vi "公式写入.vi"(7 "公式":cluster{"X^2":dbl, "X":dbl, "b":dbl}, 8 "error in (no error)":errorcluster caption="错误输入（无错误）", 9 "量程":enum16{"低量程", "高量程"}(ring), 10 "测量模式":enum16{"水样测量", "零点核查", "跨度核查", "标样核查", "加标回收"}(ring), 11 "测量参数":enum16{"总磷", "总氮", "氨氮"}(ring)) -> (0 "error out":errorcluster caption="错误输出")   [LabVIEW 2016, in "斯坦道氨氮.lvlib"]
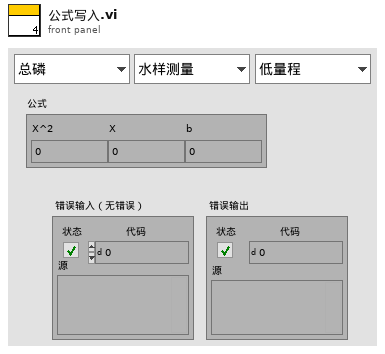
[diagram p1: front panel]
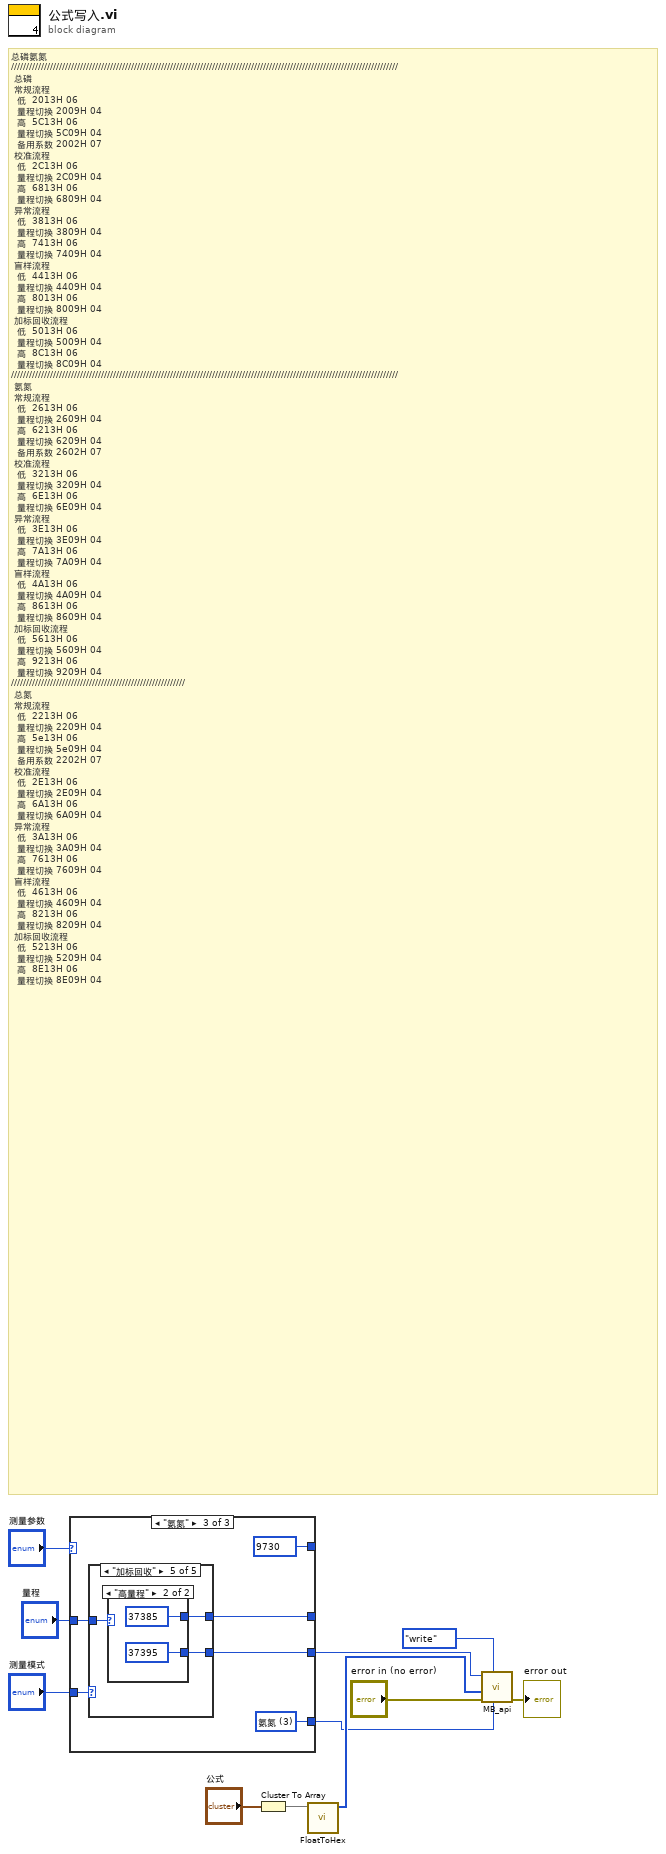
[diagram p0: block diagram]
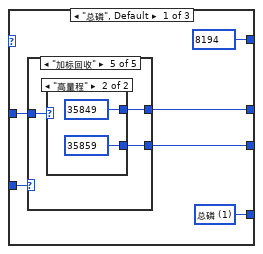
[diagram p2: hidden frame]
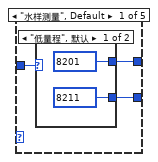
[diagram p3: hidden frame]
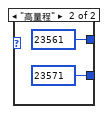
[diagram p4: hidden frame]
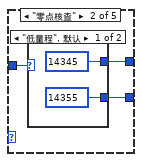
[diagram p5: hidden frame]
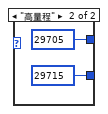
[diagram p6: hidden frame]
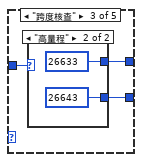
[diagram p7: hidden frame]
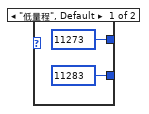
[diagram p8: hidden frame]
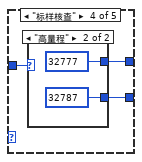
[diagram p9: hidden frame]
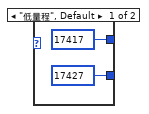
[diagram p10: hidden frame]
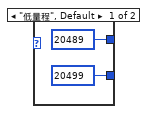
[diagram p11: hidden frame]
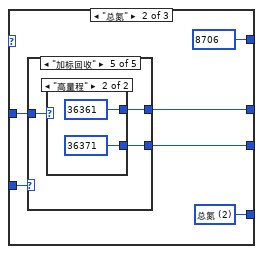
[diagram p12: hidden frame]
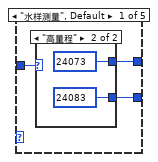
[diagram p13: hidden frame]
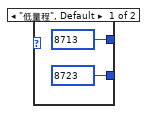
[diagram p14: hidden frame]
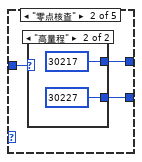
[diagram p15: hidden frame]
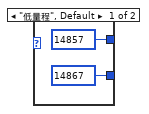
[diagram p16: hidden frame]
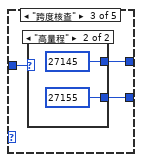
[diagram p17: hidden frame]
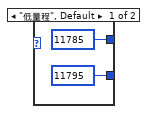
[diagram p18: hidden frame]
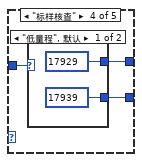
[diagram p19: hidden frame]
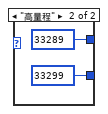
[diagram p20: hidden frame]
diagram:
  # "总磷氨氮\n/////////////////////////////////////////////////////////////////////////////////////////////////////////////////////////////////\n\t总磷\n\t常规流程\n\t\t低\t\t2013H\t06\n\t\t量程切换\t2009H\t04\n\t\t高\t\t5C13H\t06\n\t\t量程切换\t5C09H\t04\n\t\t备用系数\t2002H\t07\n\t校准流程\n\t\t低\t\t2C13H\t06\n\t\t量程切换\t2C09H\t04\n\t\t高\t\t6813H\t06\n\t\t量程切换\t6809H\t04\n\t异常流程\n\t\t低\t\t3813H\t06\n\t\t量程切换\t3809H\t04\n\t\t高\t\t7413H\t06\n\t\t量程切换\t7409H\t04\t\n\t盲样流程\n\t\t低\t\t4413H\t06\n\t\t量程切换\t4409H\t04\n\t\t高\t\t8013H\t06\n\t\t量程切换\t8009H\t04\t\n\t加标回收流程\n\t\t低\t\t5013H\t06\n\t\t量程切换\t5009H\t04\n\t\t高\t\t8C13H\t06\n\t\t量程切换\t8C09H\t04\t\n/////////////////////////////////////////////////////////////////////////////////////////////////////////////////////////////////\n\t氨氮\n\t常规流程\n\t\t低\t\t2613H\t06\n\t\t量程切换\t2609H\t04\n\t\t高\t\t6213H\t06\n\t\t量程切换\t6209H\t04\n\t\t备用系数\t2602H\t07\n\t校准流程\n\t\t低\t\t3213H\t06\n\t\t量程切换\t3209H\t04\n\t\t高\t\t6E13H\t06\n\t\t量程切换\t6E09H\t04\n\t异常流程\n\t\t低\t\t3E13H\t06\n\t\t量程切换\t3E09H\t04\n\t\t高\t\t7A13H\t06\n\t\t量程切换\t7A09H\t04\t\n\t盲样流程\n\t\t低\t\t4A13H\t06\n\t\t量程切换\t4A09H\t04\n\t\t高\t\t8613H\t06\n\t\t量程切换\t8609H\t04\t\n\t加标回收流程\n\t\t低\t\t5613H\t06\n\t\t量程切换\t5609H\t04\n\t\t高\t\t9213H\t06\n\t\t量程切换\t9209H\t04\t\n//////////////////////////////////////////////////////////\n\t总氮\n\t常规流程\n\t\t低\t\t2213H\t06\n\t\t量程切换\t2209H\t04\n\t\t高\t\t5e13H\t06\n\t\t量程切换\t5e09H\t04\n\t\t备用系数\t2202H\t07\n\t校准流程\n\t\t低\t\t2E13H\t06\n\t\t量程切换\t2E09H\t04\n\t\t高\t\t6A13H\t06\n\t\t量程切换\t6A09H\t04\n\t异常流程\n\t\t低\t\t3A13H\t06\n\t\t量程切换\t3A09H\t04\n\t\t高\t\t7613H\t06\n\t\t量程切换\t7609H\t04\t\n\t盲样流程\n\t\t低\t\t4613H\t06\n\t\t量程切换\t4609H\t04\n\t\t高\t\t8213H\t06\n\t\t量程切换\t8209H\t04\t\n\t加标回收流程\n\t\t低\t\t5213H\t06\n\t\t量程切换\t5209H\t04\n\t\t高\t\t8E13H\t06\n\t\t量程切换\t8E09H\t04"
  n1 = case shown="\"氨氮\"" "测量参数" {
    tunnel: "测量模式" -> [w17 w58 w99]
    tunnel: "量程" -> [w16 w57 w98]
    tunnel: [w15 w56 w97] -> w1
    tunnel: [w14 w55 w96] -> w8
    tunnel: [w13 w54 w95] -> _
    tunnel: [u16 8194 ("starting address") u16 8706 ("starting address") u16 9730 ("starting address")] -> _
    frame "总磷", Default {
      w15 = u16 1 items=["总磷"=1, "氨氮"=3] ("站号")
      n2 = case shown="\"加标回收\"" w17 {
        tunnel: w16 -> [w20 w27 w34 w41 w48]
        tunnel: [w19 w26 w33 w40 w47] -> w14
        tunnel: [w18 w25 w32 w39 w46] -> w13
        frame "水样测量", Default {
          n3 = case shown="\"低量程\", 默认" w20 {
            tunnel: [u16 8211 ("starting address") u16 23571 ("starting address")] -> w19
            tunnel: [u16 8201 ("starting address") u16 23561 ("starting address")] -> w18
            frame "低量程", Default {
            }
            frame "高量程" {
            }
          }
        }
        frame "零点核查" {
          n4 = case shown="\"低量程\", 默认" w27 {
            tunnel: [u16 14355 ("starting address") u16 29715 ("starting address")] -> w26
            tunnel: [u16 14345 ("starting address") u16 29705 ("starting address")] -> w25
            frame "低量程", Default {
            }
            frame "高量程" {
            }
          }
        }
        frame "跨度核查" {
          n5 = case shown="\"高量程\"" w34 {
            tunnel: [u16 11283 ("starting address") u16 26643 ("starting address")] -> w33
            tunnel: [u16 11273 ("starting address") u16 26633 ("starting address")] -> w32
            frame "低量程", Default {
            }
            frame "高量程" {
            }
          }
        }
        frame "标样核查" {
          n6 = case shown="\"高量程\"" w41 {
            tunnel: [u16 17427 ("starting address") u16 32787 ("starting address")] -> w40
            tunnel: [u16 17417 ("starting address") u16 32777 ("starting address")] -> w39
            frame "低量程", Default {
            }
            frame "高量程" {
            }
          }
        }
        frame "加标回收" {
          n7 = case shown="\"高量程\"" w48 {
            tunnel: [u16 20499 ("starting address") u16 35859 ("starting address")] -> w47
            tunnel: [u16 20489 ("starting address") u16 35849 ("starting address")] -> w46
            frame "低量程", Default {
            }
            frame "高量程" {
            }
          }
        }
      }
    }
    frame "总氮" {
      w56 = u16 2 items=["总磷"=1, "总氮"=2, "氨氮"=3] ("站号")
      n8 = case shown="\"加标回收\"" w58 {
        tunnel: w57 -> [w61 w68 w75 w82 w89]
        tunnel: [w60 w67 w74 w81 w88] -> w55
        tunnel: [w59 w66 w73 w80 w87] -> w54
        frame "水样测量", Default {
          n9 = case shown="\"高量程\"" w61 {
            tunnel: [u16 8723 ("starting address") u16 24083 ("starting address")] -> w60
            tunnel: [u16 8713 ("starting address") u16 24073 ("starting address")] -> w59
            frame "低量程", Default {
            }
            frame "高量程" {
            }
          }
        }
        frame "零点核查" {
          n10 = case shown="\"高量程\"" w68 {
            tunnel: [u16 14867 ("starting address") u16 30227 ("starting address")] -> w67
            tunnel: [u16 14857 ("starting address") u16 30217 ("starting address")] -> w66
            frame "低量程", Default {
            }
            frame "高量程" {
            }
          }
        }
        frame "跨度核查" {
          n11 = case shown="\"高量程\"" w75 {
            tunnel: [u16 11795 ("starting address") u16 27155 ("starting address")] -> w74
            tunnel: [u16 11785 ("starting address") u16 27145 ("starting address")] -> w73
            frame "低量程", Default {
            }
            frame "高量程" {
            }
          }
        }
        frame "标样核查" {
          n12 = case shown="\"低量程\", 默认" w82 {
            tunnel: [u16 17939 ("starting address") u16 33299 ("starting address")] -> w81
            tunnel: [u16 17929 ("starting address") u16 33289 ("starting address")] -> w80
            frame "低量程", Default {
            }
            frame "高量程" {
            }
          }
        }
        frame "加标回收" {
          n13 = case shown="\"高量程\"" w89 {
            tunnel: [u16 21011 ("starting address") u16 36371 ("starting address")] -> w88
            tunnel: [u16 21001 ("starting address") u16 36361 ("starting address")] -> w87
            frame "低量程", Default {
            }
            frame "高量程" {
            }
          }
        }
      }
    }
    frame "氨氮" {
      w97 = u16 3 items=["总磷"=1, "氨氮"=3] ("站号")
      n14 = case shown="\"加标回收\"" w99 {
        tunnel: w98 -> [w102 w109 w116 w123 w130]
        tunnel: [w101 w108 w115 w122 w129] -> w96
        tunnel: [w100 w107 w114 w121 w128] -> w95
        frame "水样测量", Default {
          n15 = case shown="\"高量程\"" w102 {
            tunnel: [u16 9747 ("starting address") u16 25107 ("starting address")] -> w101
            tunnel: [u16 9737 ("starting address") u16 25097 ("starting address")] -> w100
            frame "低量程", Default {
            }
            frame "高量程" {
            }
          }
        }
        frame "零点核查" {
          n16 = case shown="\"高量程\"" w109 {
            tunnel: [u16 15891 ("starting address") u16 31251 ("starting address")] -> w108
            tunnel: [u16 15881 ("starting address") u16 31241 ("starting address")] -> w107
            frame "低量程", Default {
            }
            frame "高量程" {
            }
          }
        }
        frame "跨度核查" {
          n17 = case shown="\"低量程\", 默认" w116 {
            tunnel: [u16 12819 ("starting address") u16 28179 ("starting address")] -> w115
            tunnel: [u16 12809 ("starting address") u16 28169 ("starting address")] -> w114
            frame "低量程", Default {
            }
            frame "高量程" {
            }
          }
        }
        frame "标样核查" {
          n18 = case shown="\"低量程\", 默认" w123 {
            tunnel: [u16 18963 ("starting address") u16 34323 ("starting address")] -> w122
            tunnel: [u16 18953 ("starting address") u16 34313 ("starting address")] -> w121
            frame "低量程", Default {
            }
            frame "高量程" {
            }
          }
        }
        frame "加标回收" {
          n19 = case shown="\"高量程\"" w130 {
            tunnel: [u16 22035 ("starting address") u16 37395 ("starting address")] -> w129
            tunnel: [u16 22025 ("starting address") u16 37385 ("starting address")] -> w128
            frame "低量程", Default {
            }
            frame "高量程" {
            }
          }
        }
      }
    }
  }
  n20 = Cluster To Array(cluster="公式") -> (array=w4:dbl[])
  n21 = call "FloatToHex.vi"("浮点数"=w4) -> ("DCBA整形输出"=w3:u16[])  [unwired: 10 in]
  n22 = call "MB_api.vi"("Slave ID"=w1, "STEP"=enum16{"open", "read", "write", "close"}."write", "Error in"="error in (no error)", "values"=w3, "starting address"=w8) -> ("error out"=→"error out":errorcluster)  [unwired: 4 in, 2 out]
